vi "Init Values.vi"(8 "error in (no error)":errorcluster, 11 "Server in":refnum<class "Server.lvclass">) -> (0 "error out":errorcluster, 3 "Server out":refnum<class "Server.lvclass">)   [LabVIEW 2020, in "HTTP Server.lvlib" / "Server.lvclass"]
uses:
  Server.lvclass
  Server.lvclass/Server.ctl
  340bd801-992d-45d4-9d8e-2df6e8f38c36.vi/dd2842a1-4313-49a6-90f2-c24c0bceb404.vi
  Values/_Add Argument.vi
  Values/Values.lvclass
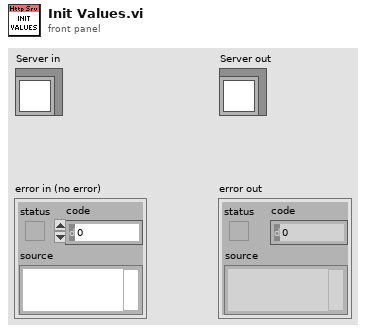
[diagram p1: front panel]
types:
  T1 = typedef "HTTP Server.lvlib/Server.lvclass/Ref Data.ctl" = cluster{"Connection Handler Map":T2, "Request Handler Map":T4, "Route Handler Map":T5, "Controller Handler Map":T6, "Controller Map":T7, "Response Handler Map":T8, "Complete Handler Map":T9, "Exception Handler Map":T10, "Connection Handler Index":u16, "Request Handler Index":u16, "Route Handler Index":u16, "Controller Handler Index":u16, "Controller Index":u16, "Response Handler Index":u16, "Complete Handler Index":u16, "Exception Handler Index":u16, "Values":refnum<class "Values.lvclass">, "Path":path, "Session Type":refnum<class "Session.lvclass">, "Session Cookie Name":string, "WebSocket Handler":refnum<class "WebSocket Handler.lvclass">, "WebSocket Handling":bool}
  T2 = typedef "HTTP Server.lvlib/Connection Handler Map.ctl" = map{T3, refnum<class "Connection Handler.lvclass">}
  T3 = typedef "HTTP Server.lvlib/Priority.ctl" = cluster{"Entity":u16, "Index":u16}
  T4 = typedef "HTTP Server.lvlib/Request Handler Map.ctl" = map{T3, refnum<class "Request Handler.lvclass">}
  T5 = typedef "HTTP Server.lvlib/Route Handler Map.ctl" = map{T3, refnum<class "Route Handler.lvclass">}
  T6 = typedef "HTTP Server.lvlib/Controller Handler Map.ctl" = map{T3, refnum<class "Controller Handler.lvclass">}
  T7 = typedef "HTTP Server.lvlib/Controller Map.ctl" = map{T3, refnum<class "Controller.lvclass">}
  T8 = typedef "HTTP Server.lvlib/Response Handler Map.ctl" = map{T3, refnum<class "Response Handler.lvclass">}
  T9 = typedef "HTTP Server.lvlib/Complete Handler Map.ctl" = map{T3, refnum<class "Complete Handler.lvclass">}
  T10 = typedef "HTTP Server.lvlib/Exception Handler Map.ctl" = map{T3, refnum<class "Exception Handler.lvclass">}
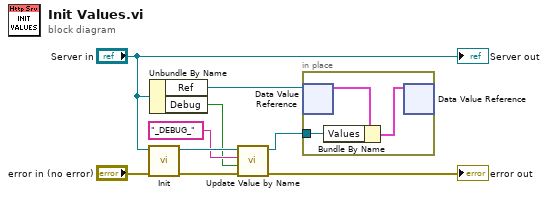
[diagram p0: block diagram]
diagram:
  n1 = call "Init.vi"("error in (no error)"="error in (no error)", "Server"="Server in") -> ("error out"=w5:errorcluster, "Arguments out"=w6:refnum<class "Values.lvclass">)  [unwired: 8 in]
  n2 = Unbundle By Name("Server in") -> ("Ref"=w8:refnum<data-value>, "Debug"=w1:bool)
  n3 = call "Update Value by Name.vi"("error in (no error)"=w5, "Value"=w1, "Name"="_DEBUG_" ("Name / Service / Object"), "Values in"=w6) -> ("error out"=→"error out":errorcluster, "Values out"=w4:refnum<class "Values.lvclass">)  [unwired: 6 in]
  n4 = in-place {
    in-place-border: w4 -> [w10]
    n5 = in-place-dvr #1(w8) -> (w12:T1)  [unwired: 1 out]
    n6 = Bundle By Name(cluster=w12, "Values"=w10) -> (w11:T1)
    n7 = in-place-dvr #1(w11) -> ()  [unwired: 2 out]
  }
  "Server out" <- "Server in"
